vi "Create FFT Plan 32f.vi"(5 "Direction":T9, 7 "FFT Types":T5, 8 "Error In":errorcluster, 9 "Dimension":T2={"Depth"=1, "Height"=1, "Width"=1} {"Width" min=1; "Height" min=1; "Depth" min=1}, 10 "FFT Dimension":T1, 11 "Labview Device":T3) -> (0 "Error Out":errorcluster, 1 "FFT Output Dimensions":T2={"Depth"=1, "Height"=1, "Width"=1} {"Width" min=1; "Height" min=1; "Depth" min=1}, 3 "FFT Object":T4 {"Imag"."Dimension"."Width" min=1; "Imag"."Dimension"."Height" min=1; "Imag"."Dimension"."Depth" min=1; "Real"."Dimension"."Width" min=1; "Real"."Dimension"."Height" min=1; "Real"."Dimension"."Depth" min=1})   [LabVIEW 2012, in "OpenCLV x64.lvlib"]
doc: "Creates a 32f FFT plan using the input values. This FFT plan stays in memory and can be re-used until destroyed. Any plan created <b>must</b> be destroyed. Allocates a memory buffer that is the proper size based on the type of FFT."
uses:
  OpenCLV x64.lvlib
  FFT Direction.ctl
  FFT Types.ctl
  FFT Control.ctl
  Controls/Device ID.ctl
  FFT Dimension.ctl
  Controls/Memory Object.ctl
  Controls/Memory ID.ctl
  User Controls/Array Dimensions.ctl
  Controls/Memory Type.ctl
  Error Checking/Add Error Functional Global.vi
  Allocate Memory/AllocateMemory_32f.vi
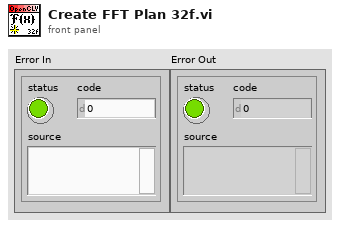
[diagram p1: front panel]
types:
  T1 = typedef "OpenCLV x64.lvlib/FFT Dimension.ctl" = enum16{"1D FFT", "2D FFT", "3D FFT"}
  T2 = typedef "Array Dimensions.ctl" = cluster{"Depth":u64, "Height":u64, "Width":u64}
  T3 = typedef "OpenCLV x64.lvlib/Device ID.ctl" = u64
  T4 = typedef "OpenCLV x64.lvlib/FFT Control.ctl" = cluster{"Device ID":T3, "FFT Types":T5, "FFT Dim":T1, "Real":T6, "Imag":T6, "FFT Plan":u64, "FFT Direction":T9}
  T5 = typedef "OpenCLV x64.lvlib/FFT Types.ctl" = enum16{"Real to Hermitian", "Hermitian to Real", "Complex to Complex"}
  T6 = typedef "OpenCLV x64.lvlib/Memory Object.ctl" = cluster{"Device ID":T3, "Memeroy ID":T7, "Dimension":T2, "Memory Type":T8}
  T7 = typedef "OpenCLV x64.lvlib/Memory ID.ctl" = u64
  T8 = typedef "OpenCLV x64.lvlib/Memory Type.ctl" = enum16{"32f", "u8", "i8", "u16", "i16", "u32", "i32", "64f"}
  T9 = typedef "OpenCLV x64.lvlib/FFT Direction.ctl" = enum16{"Forward", "Reverse"}
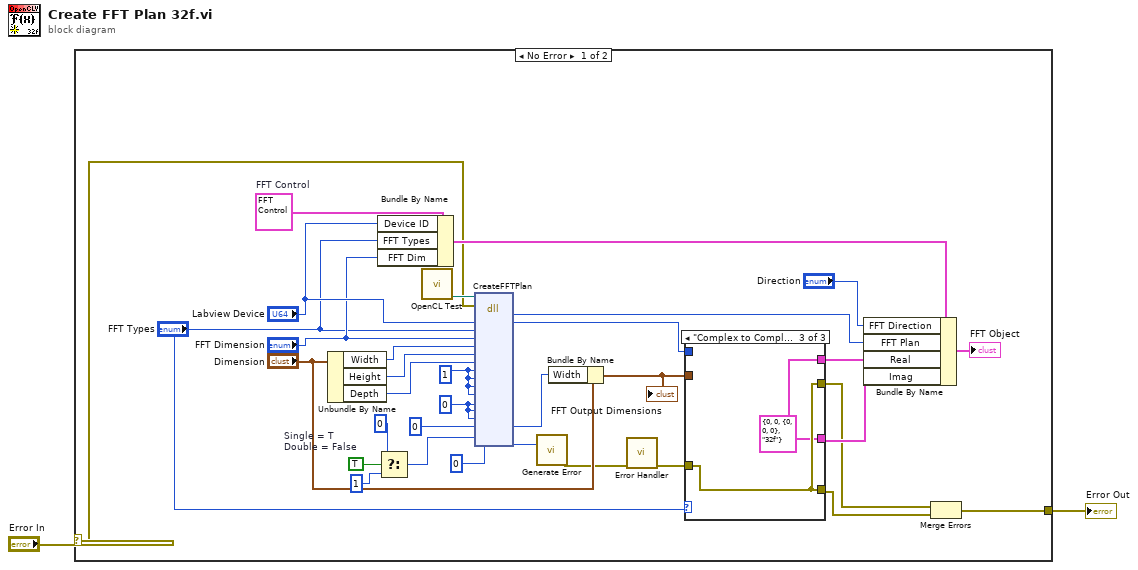
[diagram p0: block diagram]
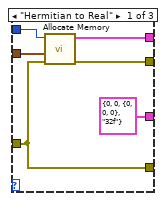
[diagram p2: hidden frame]
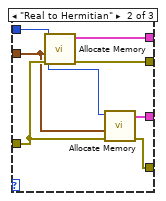
[diagram p3: hidden frame]
diagram:
  n1 = case shown="No Error" "Error In" {
    selector: "Error In" -> [w3 w51]
    tunnel: [w4 w51] -> w1
    frame No Error {
      w21 = T4 {"Device ID"=0, "FFT Types"=enum."Real to Hermitian", "FFT Dim"=enum."1D FFT", "Real"={"Device ID"=0, "Memeroy ID"=0, "Dimension"={"Depth"=0, "Height"=0, "Width"=0}, "Memory Type"=enum."32f"}, "Imag"={"Device ID"=0, "Memeroy ID"=0, "Dimension"={"Depth"=0, "Height"=0, "Width"=0}, "Memory Type"=enum."32f"}, "FFT Plan"=0, "FFT Direction"=enum."Forward"}  # FFT Control
      w33 = TRUE  # Single = T Double = False
      w26 = 0 ("StrideW")
      w25 = 1 ("StrideW")
      n2 = Unbundle By Name("Dimension") -> ("Width"=w22:u64, "Height"=w23:u64, "Depth"=w24:u64)
      n3 = Bundle By Name(cluster=w21, "Device ID"="Labview Device", "FFT Types"="FFT Types", "FFT Dim"="FFT Dimension") -> (w18:T4)
      n4 = Select(t=0, s=w33, f=1 ("t")) -> (s? t:f=w32:i32)
      n5 = call "OpenCL Test.vi"() -> ("DLL To Use"=w7:path)  [unwired: 11 in]
      n6 = dll-call lib="C:/Users/bme-amcelroy-la/Desktop/OpenCLV/trunk/OpenCLV_x64_1.0/OpenCLV_x64.dll" fn="CreateFFTPlan"(path in=w7, error in=w3, "Labview Device"="Labview Device", "FFT Type"="FFT Types", "FFT Dimensions"="FFT Dimension", "Width"=w22, "Height"=w23, "Depth"=w24, "StrideW"=w25, "StrideH"=w25, "StrideD"=w25, "StrideT"=w25, "PaddingW"=w26, "PaddingH"=w26, "PaddingD"=w26, "Output Width"=u64 0 ("BufferSize"), "SingleOrDouble"=w32, "Error"=0) -> ("FFT Plan"=w16:u64, "Labview Device"=w9:u64, "Output Width"=w31:u64, "Error"=w29:i32)  [unwired: 14 in, 2 out]
      n7 = call "Generate Error.vi"("Error"=w29) -> ("error out"=w6:errorcluster)  [unwired: 10 in]
      n8 = Bundle By Name(cluster="Dimension", "Width"=w31) -> (w10:T2)
      "FFT Output Dimensions" <- w10
      n9 = call-poly "Error Handler.vi"("Error In"=w6) -> ("Error Out"=w5:errorcluster)  [unwired: 10 in]
      n10 = case shown="\"Complex to Complex\"" "FFT Types" {
        tunnel: [w37 w48 w50] -> w11
        tunnel: [w41 w47 w50] -> w12
        tunnel: w5 -> [w37 w46 w50]
        tunnel: w10 -> [w40 w45 _]
        tunnel: [w39 w44 w49] -> w14
        tunnel: [T6 {"Device ID"=0, "Memeroy ID"=0, "Dimension"={"Depth"=0, "Height"=0, "Width"=0}, "Memory Type"=enum."32f"} ("Memory Object") w43 w49] -> w13
        tunnel: w9 -> [w38 w42 _]
        frame "Hermitian to Real" {
          n11 = call-poly "Allocate Memory.vi"("Error In"=w37, "Dimension"=w40, "Device In"=w38) -> ("Error Out"=w41:errorcluster, "Memory Object"=w39:T6)  [unwired: 6 in, 1 out]
        }
        frame "Real to Hermitian" {
          n12 = call-poly "Allocate Memory.vi"("Error In"=w46, "Dimension"=w45, "Device In"=w42) -> ("Error Out"=w47:errorcluster, "Memory Object"=w44:T6)  [unwired: 6 in, 1 out]
          n13 = call-poly "Allocate Memory.vi"("Error In"=w46, "Dimension"=w45, "Device In"=w42) -> ("Error Out"=w48:errorcluster, "Memory Object"=w43:T6)  [unwired: 6 in, 1 out]
        }
        frame "Complex to Complex" {
          w49 = T6 {"Device ID"=0, "Memeroy ID"=0, "Dimension"={"Depth"=0, "Height"=0, "Width"=0}, "Memory Type"=enum."32f"} ("Memory Object")
        }
      }
      n14 = Bundle By Name(cluster=w18, "FFT Direction"="Direction", "FFT Plan"=w16, "Real"=w14, "Imag"=w13) -> (→"FFT Object":T4)
      n15 = Merge Errors(w12, w11) -> (w4:errorcluster)
    }
    frame Error {
    }
  }
  "Error Out" <- w1
